vi "fft.vi"() -> ()   [LabVIEW 2017]
uses:
  <vilib>/Utility/file.llb/Read Delimited Spreadsheet (I64).vi
  <vilib>/addons/Digital Filter Design/CodeGen.llb/DFD FXP C Code Generator.vi
  <vilib>/addons/Digital Filter Design/Process.llb/DFD Filtering (Wfm).vi
  <vilib>/express/express analysis/Spectral/Block/exnSpectralBlock spectral measurements peak poly.vi
  <vilib>/express/express analysis/Spectral/Block/exnSpectralBlock spectral measurements peak WFM.vi
  <vilib>/express/express analysis/Spectral/Block/exnSpectralBlock spectral measurements RMS poly.vi
  <vilib>/express/express analysis/Spectral/Block/exnSpectralBlock spectral measurements RMS WFM.vi
  <vilib>/express/express analysis/Spectral/XNode/ExpressSpectralMeasurementsBlockNode.xnode
  <vilib>/addons/Digital Filter Design/FXPModel.llb/DFD FXP Quantize Coef (Easy).vi
  <vilib>/addons/Digital Filter Design/NI_DigFilterLicensed.lvlib
panel:
  in  "输出滤波C文件":bool
  out "Error Message":string
  in  "Cut-Off Frequency (Hz)":dbl(slide)=100.0 scale=10.0..17000.0
  in  "停止":bool
  out "PC 滤波后的 FFT":cluster{"f0":dbl, "df":dbl, "magnitude":dbl[]}(graph)
  out "PC滤波后的信号":waveform(dbl)(graph) caption="PC 滤波后"
  out "子数组":i64[](array[numeric])
  out "all rows":i64[][](array[numeric]) caption="所有行"
  out "原始信号FFT":cluster{"f0":dbl, "df":dbl, "magnitude":dbl[]}(graph)
  out "原始信号波形":waveform(i64)(graph) caption="原始信号"
  # "两阶高级IIR低通滤波器"
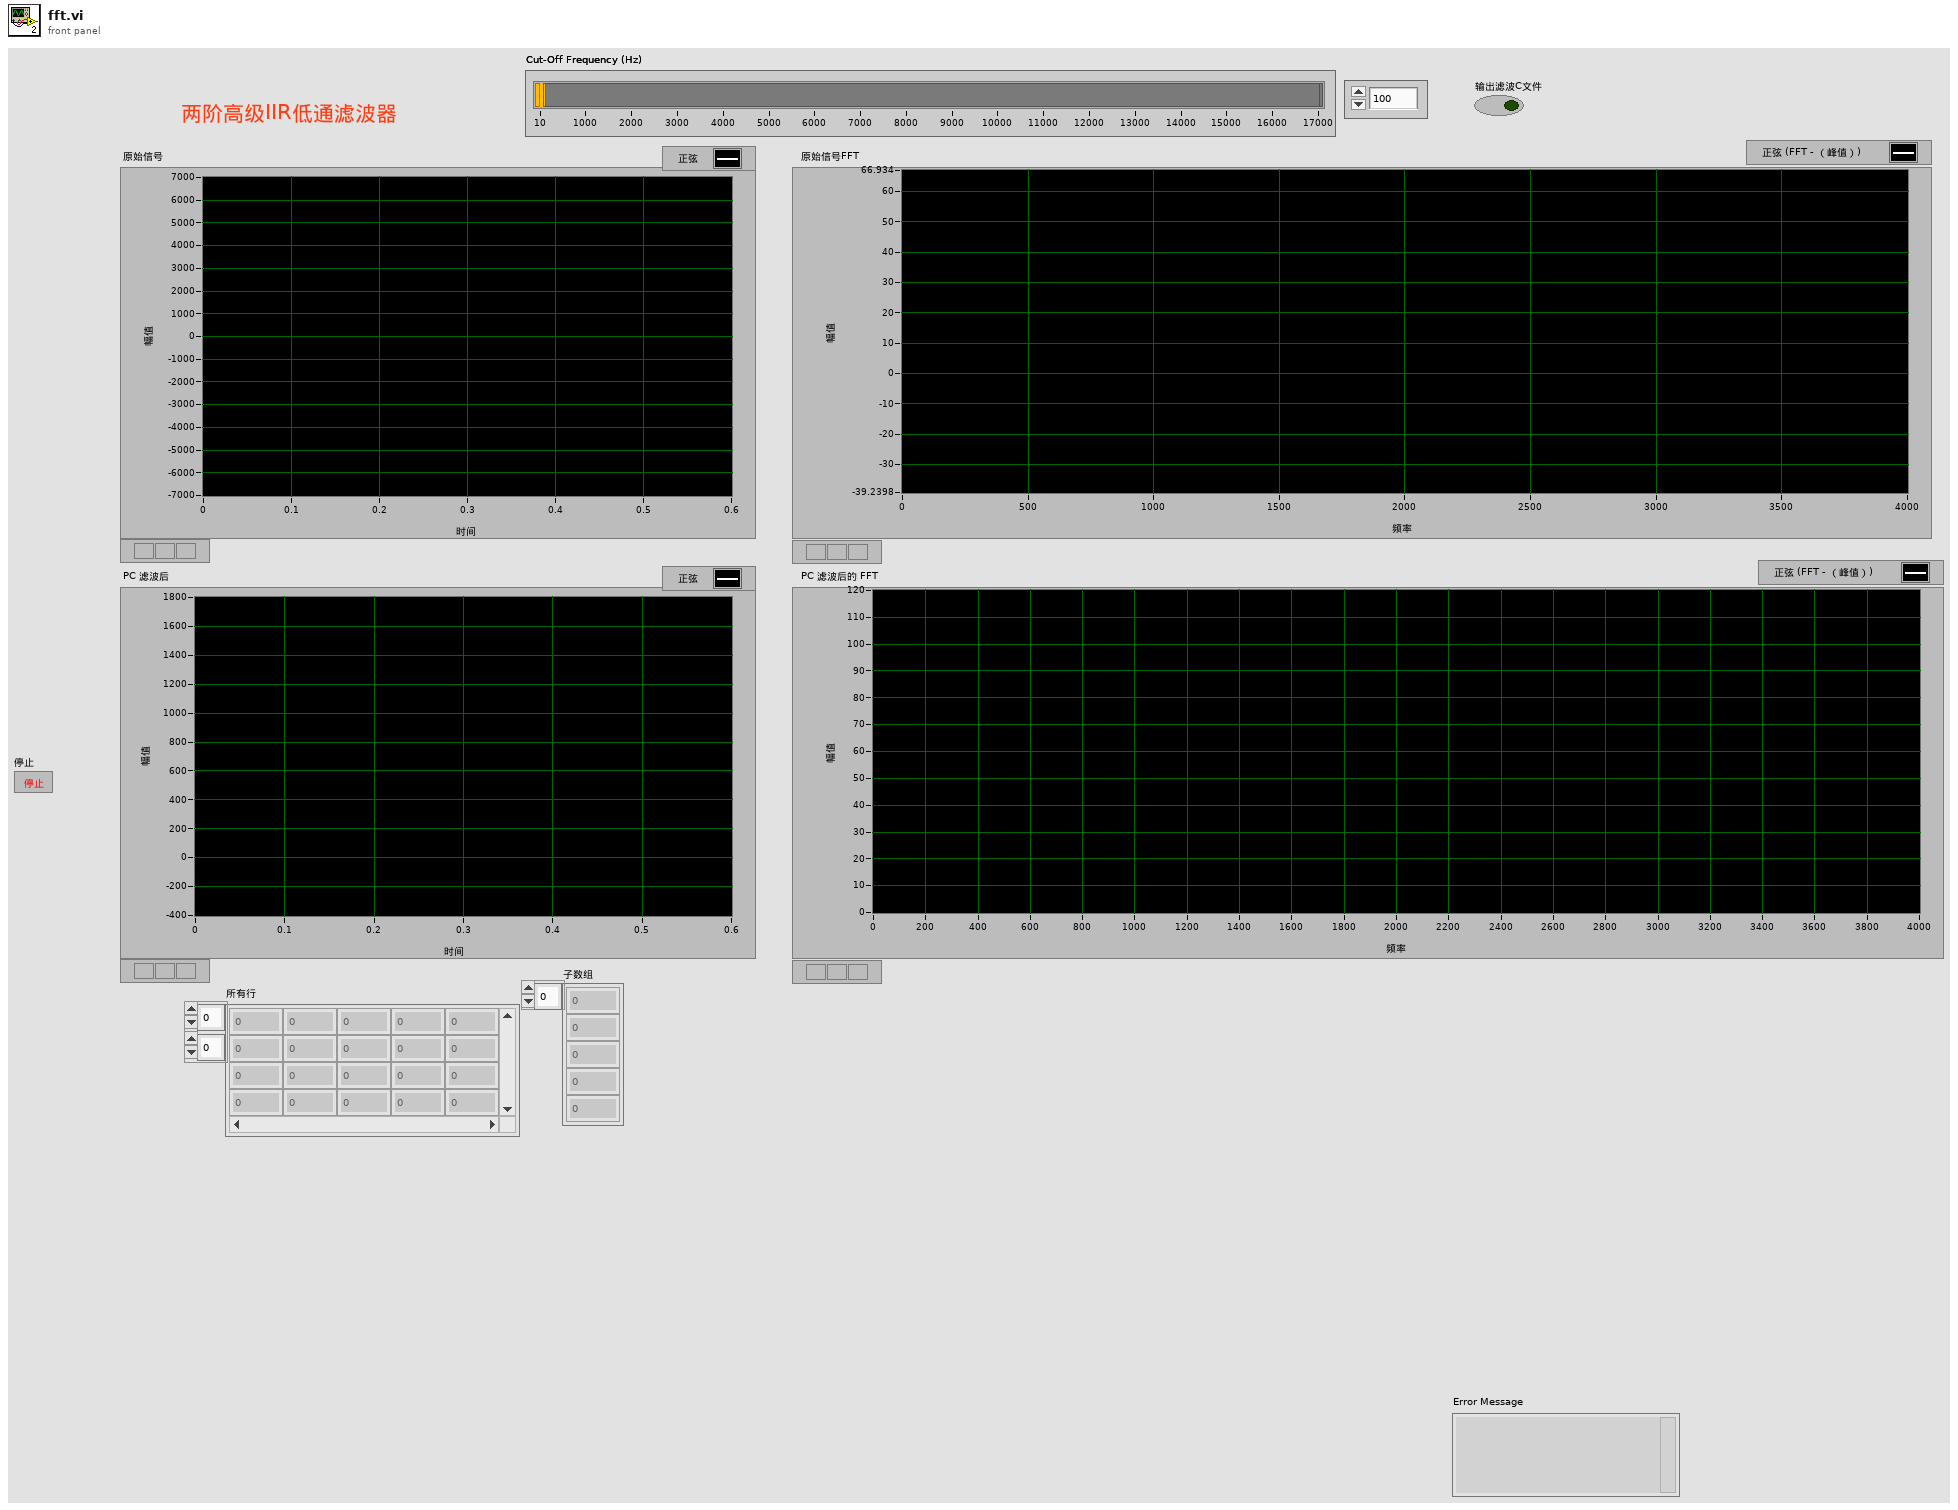
[diagram p1: front panel]
types:
  T1 = enum16{"Lowpass", "Highpass", "Bandpass", "Bandstop"}
  T2 = cluster{"averaging mode":u16, "weighting mode":u16, "number of averages":u32}
  T3 = cluster{"dB On (F)":bool, "unwrap phase (F)":bool, "convert to degree (F)":bool}
  T4 = typedef "NI_DigFilterLicensed.lvlib/DFD Filter Obj.ctl" = cluster{"mSRate_Fs":dbl, "mSRate_Version":string, "mSRate_Comments":string, "mSRate_OrgCoef":T5, "mSRate_CurCoef":T5, "mSRate_Quantized?":bool, "mSRate_QCoef":T5, "mSRate_QSettings":T7[], "mSRate_Order":i32, "mSRate_Scaling":cluster{"mSRate_ScaleByPowerOf2?":bool, "mSRate_ScaleType":T9}}
  T5 = typedef "NI_DigFilterLicensed.lvlib/DFD Filter Coef.ctl" = cluster{"type":T6, "gain":dbl, "coef a (k)":dbl[], "coef b (v)":dbl[]}
  T6 = typedef "NI_DigFilterLicensed.lvlib/DFD Filter Structure Type Selector.ctl" = enum16{"Undefined", "FIR Direct Form", "FIR Direct Form Transposed", "FIR Symmetric", "FIR Antisymmetric", "IIR Direct Form I", "IIR Direct Form I Transposed", "IIR Direct Form II", "IIR Direct Form II Transposed", "IIR Cascaded Second Order Sections Form I", "IIR Cascaded Second Order Sections Form I Transposed", "IIR Cascaded Second Order Sections Form II", "IIR Cascaded Second Order Sections Form II Transposed", "Lattice Allpass (basic sections)", "Lattice Allpass (one multiplier sections)", "Lattice Allpass (normalized sections)", "Lattice AR (basic sections)", "Lattice AR (one multiplier sections)", "Lattice AR (normalized sections)", "Lattice MA (minimum phase)", "Lattice MA (maximum phase)", "Lattice ARMA (basic sections)", "Lattice ARMA (one multiplier sections)", "Lattice ARMA (normalized sections)"}
  T7 = typedef "NI_DigFilterLicensed.lvlib/dfd_Internal Quantization Settings.ctl" = cluster{"source":T8, "wl":i16, "iwl":i16, "overflow mode":enum16{"Saturation", "Wrap"}, "rounding mode":enum16{"Nearest", "Truncation"}, "signed?":bool}
  T8 = typedef "NI_DigFilterLicensed.lvlib/dfd_Internal Quantization Srcs.ctl" = u16
  T9 = typedef "NI_DigFilterLicensed.lvlib/DFD Coef Norm Type.ctl" = enum16{"No Norm", "Time Domain 1-Norm", "Time Domain 2-Norm", "Time Domain Inf-Norm"}
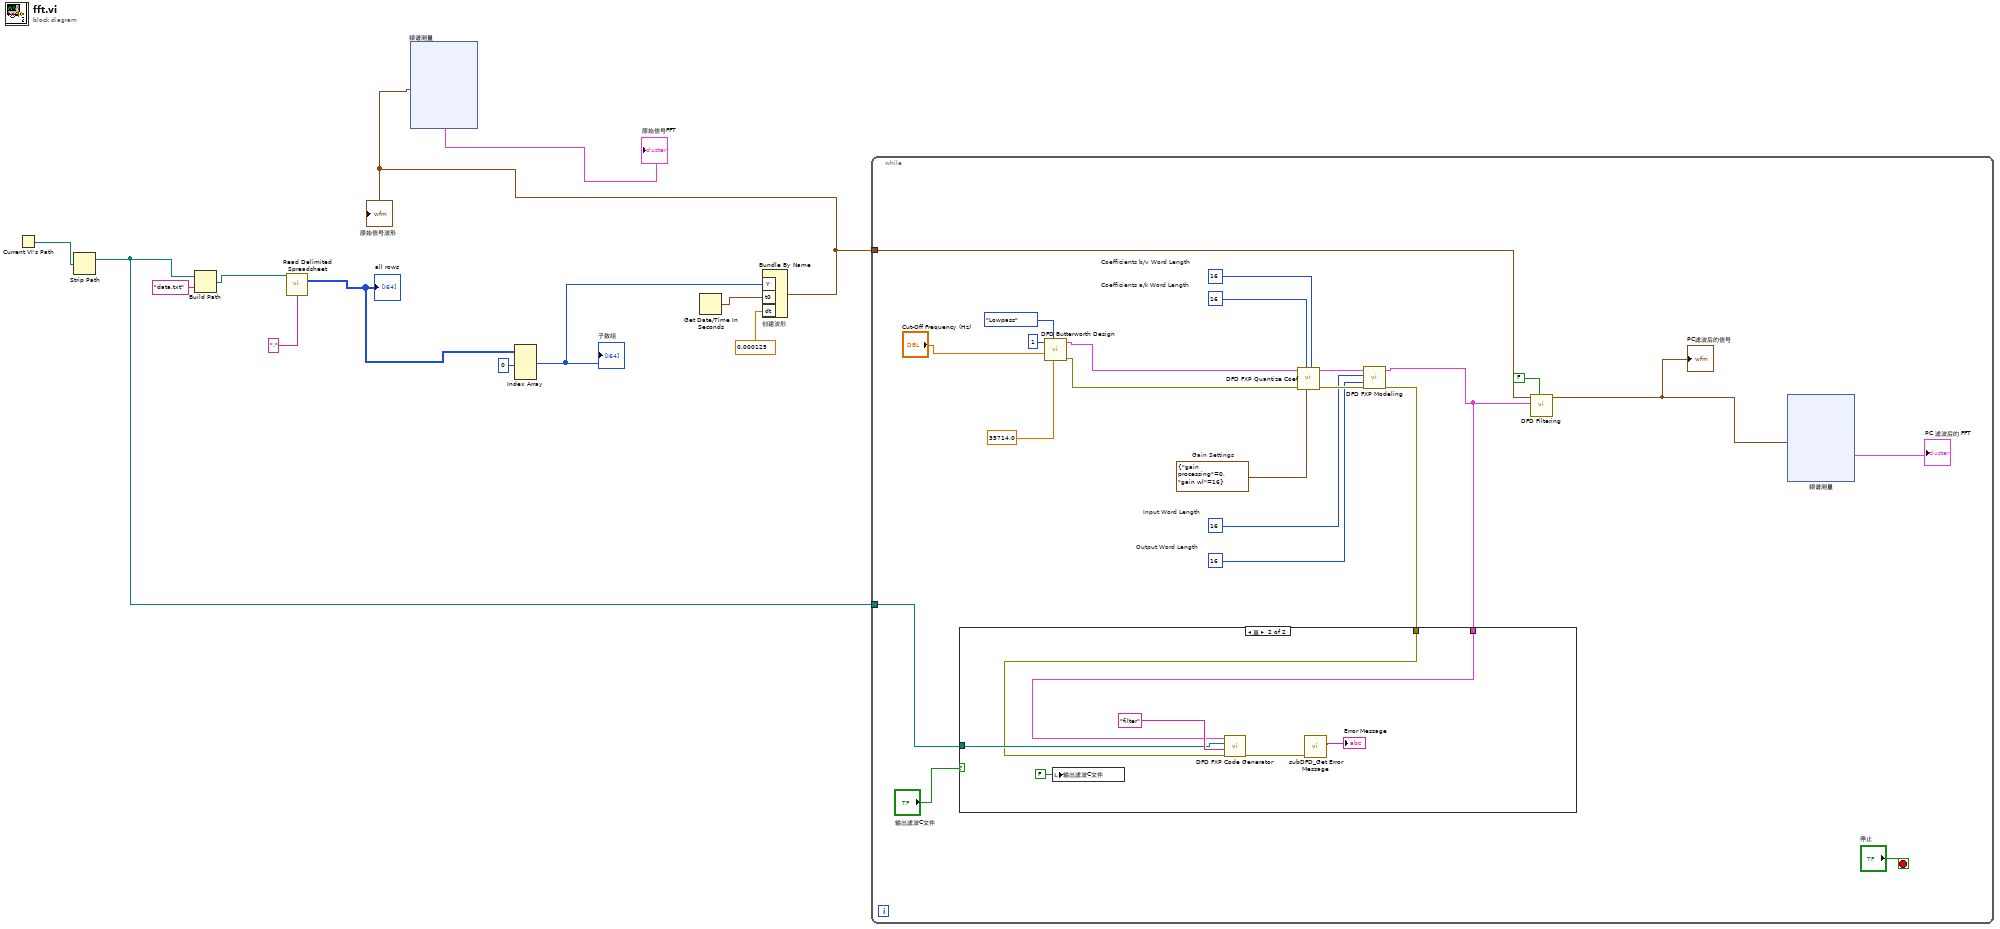
[diagram p0: block diagram]
diagram:
  n1 = Current VI's Path() -> (path=w8:path)
  n2 = Strip Path(path=w8) -> (stripped path=w5:path)  [unwired: 1 out]
  n3 = Build Path(base path=w5, name or relative path="data.txt" ("名称或相对路径")) -> (appended path=w6:path)
  n4 = call-poly <vilib>:"Read Delimited Spreadsheet.vi"("file path (dialog if empty)"=w6, "delimiter (\\t)"=",") -> ("all rows"=w10:i64[][])  [unwired: 8 in, 5 out]
  "all rows" <- w10
  n5 = Index Array(array=w10, index (col) #1=0 ("禁用的索引 (列)")) -> (element #1=w2:i64[])  [unwired: 3 in, 1 out]
  "子数组" <- w2
  n6 = Get Date/Time In Seconds() -> (seconds since 1Jan1904=w4:timestamp)
  n7 = Bundle By Name "创建波形"("Y"=w2, "t0"=w4, "dt"=0.000125) -> (w1:waveform(i64))  [unwired: 1 in]
  "原始信号波形" <- w1
  n8 = xnode "频谱测量"("信号"=w1) -> ("FFT - （均方根）"=→"原始信号FFT":cluster{"f0":dbl, "df":dbl, "magnitude":dbl[]})  [unwired: 1 in, 2 out]
  n9 = while {
    tunnel: w1 -> [w33]
    tunnel: w5 -> [w26]
    stop <- "停止" stop-if-true
    w17 = i16 16  # Coefficients b/v Word Length
    w16 = i16 16  # Coefficients a/k Word Length
    w20 = i16 16  # Output Word Length
    w21 = i16 16  # Input Word Length
    w24 = cluster{"gain processing":u16, "gain wl":i16} {"gain processing"=0, "gain wl"=16}  # Gain Settings
    n10 = call <vilib>:"DFD Butterworth Design.vi"("fs [Hz]"=35714.0, "filter type"=T1."Lowpass", "low cutoff freq [Hz]"="Cut-Off Frequency (Hz)", "order"=1) -> ("error out"=w19:errorcluster, "filter out"=w18:T4)  [unwired: 6 in]
    n11 = call-poly <vilib>:"DFD FXP Quantize Coef.vi"("coefficients b/v word length"=w17, "gain settings"=w24, "coefficients a/k word length"=w16, "error in (no error)"=w19, "filter in"=w18) -> ("error out"=w22:errorcluster, "filter out"=w23:T4)  [unwired: 5 out]
    n12 = call <vilib>:"DFD FXP Modeling.vi"("error in (no error)"=w22, "output word length"=w20, "input word length"=w21, "filter in"=w23) -> ("error out"=w15:errorcluster, "filter out"=w14:T4)  [unwired: 3 in, 3 out]
    n13 = case shown="真" "输出滤波C文件" {
      tunnel: w26 -> [_ w38]
      tunnel: w15 -> [_ w36]
      tunnel: w14 -> [_ w35]
      frame False {
      }
      frame True {
        n14 = local write "输出滤波C文件"(FALSE ("输出滤波C文件")) -> ()
        n15 = call-poly <vilib>:"DFD FXP Code Generator.vi"("error in (no error)"=w36, "filter name"="filter" ("Filter Name"), "destination folder"=w38, "filter in"=w35) -> ("error out"=w40:errorcluster)  [unwired: 3 in, 4 out]
        n16 = call <vilib>:"subDFD_Get Error Message.vi"("error in (no error)"=w40) -> ("Error Message"=→"Error Message":string)  [unwired: 10 out]
      }
    }
    n17 = call-poly <vilib>:"DFD Filtering.vi"("init? (F)"=FALSE, "filter"=w14, "signal in"=w33) -> ("signal out"=w32:waveform(dbl))  [unwired: 1 in, 7 out]
    "PC滤波后的信号" <- w32
    n18 = xnode "频谱测量"("信号"=w32) -> ("FFT - （峰值）"=→"PC 滤波后的 FFT":cluster{"f0":dbl, "df":dbl, "magnitude":dbl[]})  [unwired: 1 in, 2 out]
  }
